vi "ConvertNumericSetpointToHex.vi"(11 "Numeric Setpoint (C)":dbl format="%.1f") -> (3 "Hex Setpoint (C)":string)   [LabVIEW 2012, in "Omega-CSi32.lvlib"]
uses:
  Omega-CSi32.lvlib
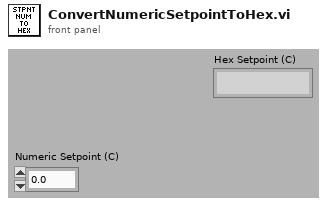
[diagram p1: front panel]
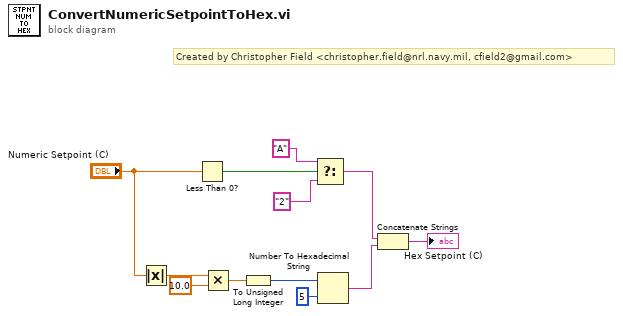
[diagram p0: block diagram]
diagram:
  # "Created by Christopher Field <christopher.field@nrl.navy.mil, cfield2@gmail.com>"
  n1 = Absolute Value(x="Numeric Setpoint (C)") -> (abs(x)=w10:dbl)
  n2 = Less Than 0?(x="Numeric Setpoint (C)") -> (x < 0?=w5:bool)
  n3 = Multiply(x=w10, y=10.0) -> (x*y=w9:dbl)
  n4 = To Unsigned Long Integer(number=w9) -> (unsigned 32bit integer=w8:u32)
  n5 = Select(t="A" ("string"), s=w5, f="2" ("string")) -> (s? t:f=w2:string)
  n6 = Number To Hexadecimal String(1:i16 5 ("width (-)"), 2:w8) -> (0:w6:string)
  n7 = Concatenate Strings(w2, w6) -> (→"Hex Setpoint (C)":string)
